vi "create IMAQ references.vi"(8 "error in (no error)":errorcluster, 11 "LineCCD in":refnum<class "LineCCD.lvclass">) -> (0 "error out":errorcluster, 3 "LineCCD out":refnum<class "LineCCD.lvclass">)   [LabVIEW 2012, in "LineCCD.lvclass"]
uses:
  LineCCD.lvclass
  LineCCD.lvclass/LineCCD.ctl
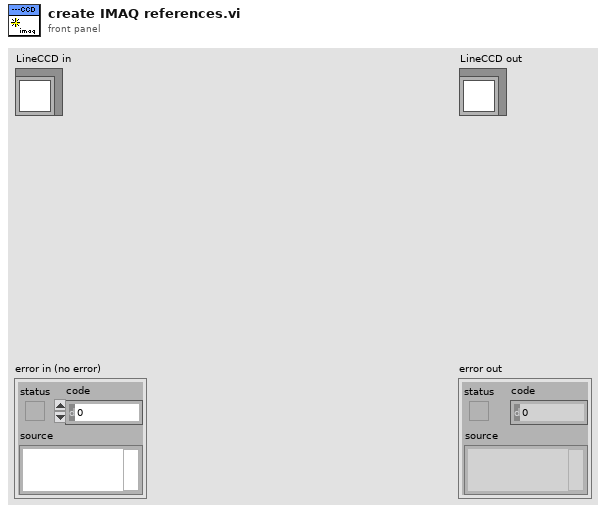
[diagram p1: front panel]
types:
  T1 = typedef "Image Type" = u32
  T2 = typedef "IMAQ Image.ctl" = refnum<image>
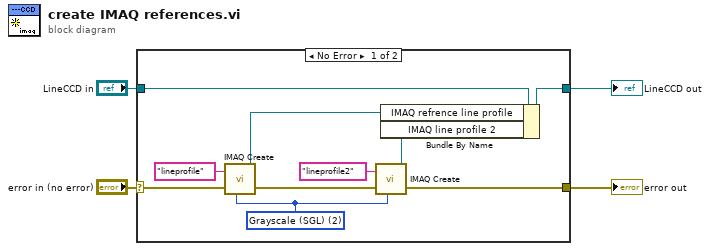
[diagram p0: block diagram]
diagram:
  n1 = case shown="No Error" "error in (no error)" {
    selector: "error in (no error)" -> [w14 w16]
    tunnel: [w5 w16] -> w3
    tunnel: [w11 w15] -> w1
    tunnel: "LineCCD in" -> [w12 w15]
    frame No Error {
      w8 = T1 2 items=["Grayscale (U8)", "Grayscale (I16)", "Grayscale (SGL)", "Complex (CSG)", "RGB (U32)", "HSL (U32)", "RGB (U64)", "Grayscale (U16)"] ("Image Type")
      n2 = call "IMAQ Create"("Image Name"="lineprofile", "Image Type"=w8, "error in (no error)"=w14) -> ("New Image"=w7:T2, "error out"=w9:errorcluster)  [unwired: 2 in]
      n3 = call "IMAQ Create"("Image Name"="lineprofile2", "Image Type"=w8, "error in (no error)"=w9) -> ("New Image"=w6:T2, "error out"=w5:errorcluster)  [unwired: 2 in]
      n4 = Bundle By Name(cluster=w12, "IMAQ refrence line profile"=w7, "IMAQ line profile 2"=w6) -> (w11:refnum<class "LineCCD.lvclass">)
    }
    frame Error {
    }
  }
  "error out" <- w3
  "LineCCD out" <- w1
